vi "Configure Serial Bus (Flexray - Trigger - Error).vi"(0 "VISA resource name":refnum<visa-resource-name>, 5 "Serial Bus Name (1: Serial Bus 1)":i32(ring)=1 items=["Serial Bus 1"=1, "Serial Bus 2"=2], 9 "Error Type (0: ALL)":i32(ring) items=["All", "Header CRC", "Frame CRC"], 11 "error in (no error)":errorcluster) -> (4 "VISA resource name out":refnum<visa-resource-name>, 15 "error out":errorcluster)   [LabVIEW 2016, in "Agilent 2000 3000 X-Series.lvlib"]
doc: "Configures the Error Trigger settings of FlexRay bus. The event setting is only valid when the FlexRay trigger mode is set to Error."
uses:
  Agilent 2000 3000 X-Series.lvlib
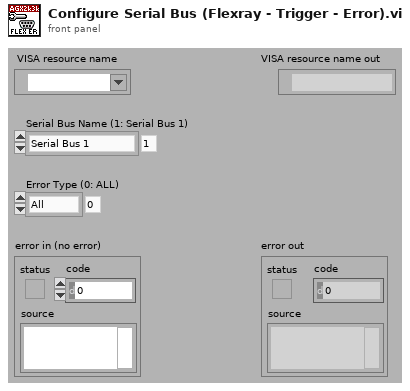
[diagram p1: front panel]
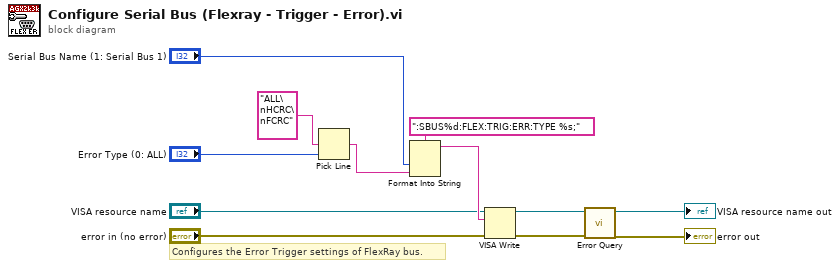
[diagram p0: block diagram]
diagram:
  # "Configures the Error Trigger settings of FlexRay bus."
  n1 = Pick Line(multi-line string="ALL\nHCRC\nFCRC", line index="Error Type (0: ALL)") -> (output string=w8:string)  [unwired: 1 out]
  n2 = Format Into String(format string=":SBUS%d:FLEX:TRIG:ERR:TYPE %s;", "Serial Bus Name (1: Serial Bus 1)", w8) -> (resulting string=w7:string)  [unwired: 2 in, 1 out]
  n3 = VISA Write(VISA resource name="VISA resource name", write buffer=w7, error in (no error)="error in (no error)") -> (VISA resource name out=w4:refnum<visa-resource-name>, error out=w3:errorcluster)  [unwired: 1 out]
  n4 = call "Error Query.vi"("error in (no error)"=w3, "VISA resource name"=w4) -> ("error out"=→"error out":errorcluster, "VISA resource name out"=→"VISA resource name out":refnum<visa-resource-name>)  [unwired: 8 out]
